vi "2L10_OBS_ou_MIF.vi"(1 "ni":u32[](array[numeric])) -> (0 "OBS/MIF":enum16{"OBS", "MIF"}(ring))   [LabVIEW 2010, in "lv_02.lvlib"]
uses:
  lv_02.lvlib
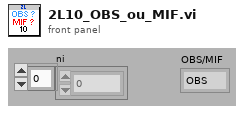
[diagram p1: front panel]
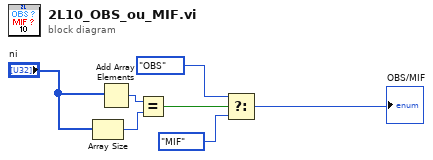
[diagram p0: block diagram]
diagram:
  n1 = Array Size(array="ni") -> (size(s)=w5:i32)
  n2 = Add Array Elements(numeric array="ni") -> (sum=w4:u32)
  n3 = Equal?(x=w4, y=w5) -> (x = y?=w7:bool)
  n4 = Select(t=enum16{"OBS", "MIF"}."OBS" ("Obs. 2"), s=w7, f=enum16{"OBS", "MIF"}."MIF" ("Obs. 2")) -> (s? t:f=→"OBS/MIF":enum16{"OBS", "MIF"})
